vi "VIRCdll.vi"(8 "error in (no error)":errorcluster, 10 "z":dbl[](array[numeric]), 11 "t":dbl) -> (0 "error out":errorcluster, 3 "ca out":dbl)   [LabVIEW 2015]
doc: "subroutine VIRC (t,z,ca)\n\nCompute the third virial coefficient as a function of temperature and composition.\n\nINPUTS:\n t--temperature [K]\n z--composition [array of mol frac]\n\nOUTPUTS:\n ca--third virial coefficient [(L/mol)^2]"
uses:
  REFPROP.dll
panel:
  # "REFPROP-VIRCdll.vi"
  # "void  VIRCdll(double *t, double *z, double *ca);"
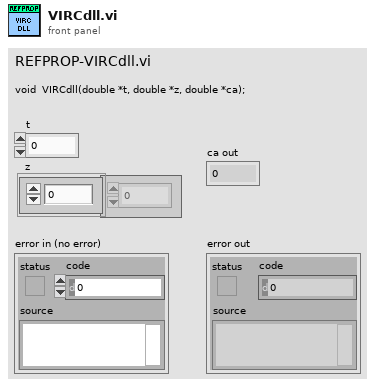
[diagram p1: front panel]
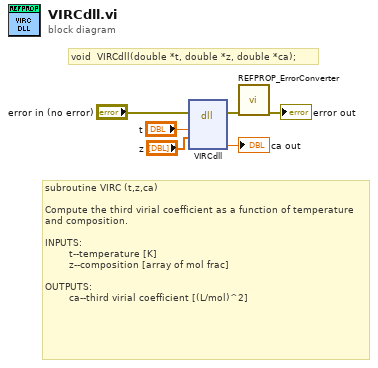
[diagram p0: block diagram]
diagram:
  # "void  VIRCdll(double *t, double *z, double *ca);"
  # "subroutine VIRC (t,z,ca)\n\nCompute the third virial coefficient as a function of temperature and composition.\n\nINPUTS:\n        t--temperature [K]\n        z--composition [array of mol frac]\n\nOUTPUTS:\n        ca--third virial coefficient [(L/mol)^2]"
  n1 = dll-call lib="C:/Users/lauria/Desktop/REFPROP 10 LabVIEW Wrapper BETA/REFPROP/REFPROP.*" fn="VIRCdll"(error in="error in (no error)", "t"="t", "z"="z") -> (error out=w3:errorcluster, "ca"=→"ca out":dbl)  [unwired: 6 in, 1 out]
  n2 = call "REFPROP_ErrorConverter.vi"("error in (no error)"=w3) -> ("error out"=→"error out":errorcluster)  [unwired: 10 in]
